vi "Generate 2D scan Waveform.vi"() -> ()   [LabVIEW 2014]
uses:
  <vilib>/Analysis/NI_AALBase.lvlib
  <vilib>/Analysis/1siggen.llb/Ramp Pattern by Samples.vi
  Controls/Translation Stage Types.ctl
  Hardware/Table Stage/Controls/Translation Stage Cluster.ctl
  Controls/System Parameters.ctl
panel:
  out "XY Graph":cluster{"X":dbl, "Y":dbl}[](graph)
  out "um/px":dbl
  in  "System Parameters [In]":T1={"Optical /HW Parameters"={"Focal Length [mm]"=0.0, "Scan Lens EFL[mm]"=0.0, "Tube Lens EFL[mm]"=0.0, "Galvo V Range (+/-)"=0.0, "Galvo Max Half Angle [Deg]"=0.0, "Max Galvo Range[%]"=0.0}, "Vibratome"={"Z Bottom [mm]"=0.0, "Pre Cut Dwell [s]"=0.0, "Blade Frequency [RPM]"=0, "Slice Speed [mm/s]"=0.0, "Post Cut Dwell [s]"=0.0, "Ramp Time [s]"=0.0, "Start X [mm]"=0.0, "Start Y [mm]"=0.0, "Slice Length [mm]"=0.0, "Slice Axis"=enum."Y Axis", "Controller VISA Ref"="COM4"}, "Table Stages"={"X Stage"={"Position"=0.0, "Is.Enabled?"=FALSE, "Is.Connected?"=FALSE, "Device SN"="45876539", "AccelerationMaximum"=0.0, "VelocityMaximum"=0.0, "Acceleration"=0.0, "Velocity"=0.0, "waitTimeout (ms)"=0, "Model"=enum."None", "Is.Homed?"=FALSE}, "Y Stage"={"Position"=0.0, "Is.Enabled?"=FALSE, "Is.Connected?"=FALSE, "Device SN"="45876539", "AccelerationMaximum"=0.0, "VelocityMaximum"=0.0, "Acceleration"=0.0, "Velocity"=0.0, "waitTimeout (ms)"=0, "Model"=enum."None", "Is.Homed?"=FALSE}, "Z Stage"={"Position"=0.0, "Is.Enabled?"=FALSE, "Is.Connected?"=FALSE, "Device SN"="45876539", "AccelerationMaximum"=0.0, "VelocityMaximum"=0.0, "Acceleration"=0.0, "Velocity"=0.0, "waitTimeout (ms)"=0, "Model"=enum."None", "Is.Homed?"=FALSE}}, "Imaging Parameter"={"Pixel Dwell Time [ms]"=0.0, "XY Center [um]"={"X"=1.0, "Y"=1.0}, "Zoom Factor"=1.0, "Display Channel"=enum."Channel A", "XY Image Resolution"=enum."256 x 256", "Custom"=FALSE, "Custom Size"={"X"=1, "Y"=1}, "Averaging"={"A Frame Ave."=1, "B Frame Ave."=1, "C Frame Ave. "=1}}} {"Imaging Parameter"."Custom Size"."Y" min=1 max=30 step=1; "Imaging Parameter"."Custom Size"."X" min=1 max=30 step=1; "Imaging Parameter"."XY Center [um]"."Y" min=1.0 max=30.0 step=1.0; "Imaging Parameter"."XY Center [um]"."X" min=1.0 max=30.0 step=1.0; "Imaging Parameter"."Averaging"."C Frame Ave." min=1 max=30 step=1; "Imaging Parameter"."Averaging"."B Frame Ave." min=1 max=30 step=1; "Imaging Parameter"."Averaging"."A Frame Ave." min=1 max=30 step=1; "Imaging Parameter"."Zoom Factor" min=1.0 max=10.0 step=0.1 scale=1.0..30.0; "Imaging Parameter"."Pixel Dwell Time [ms]" min=0.0 max=10.0 step=0.01}
  # "X"
  # "X"
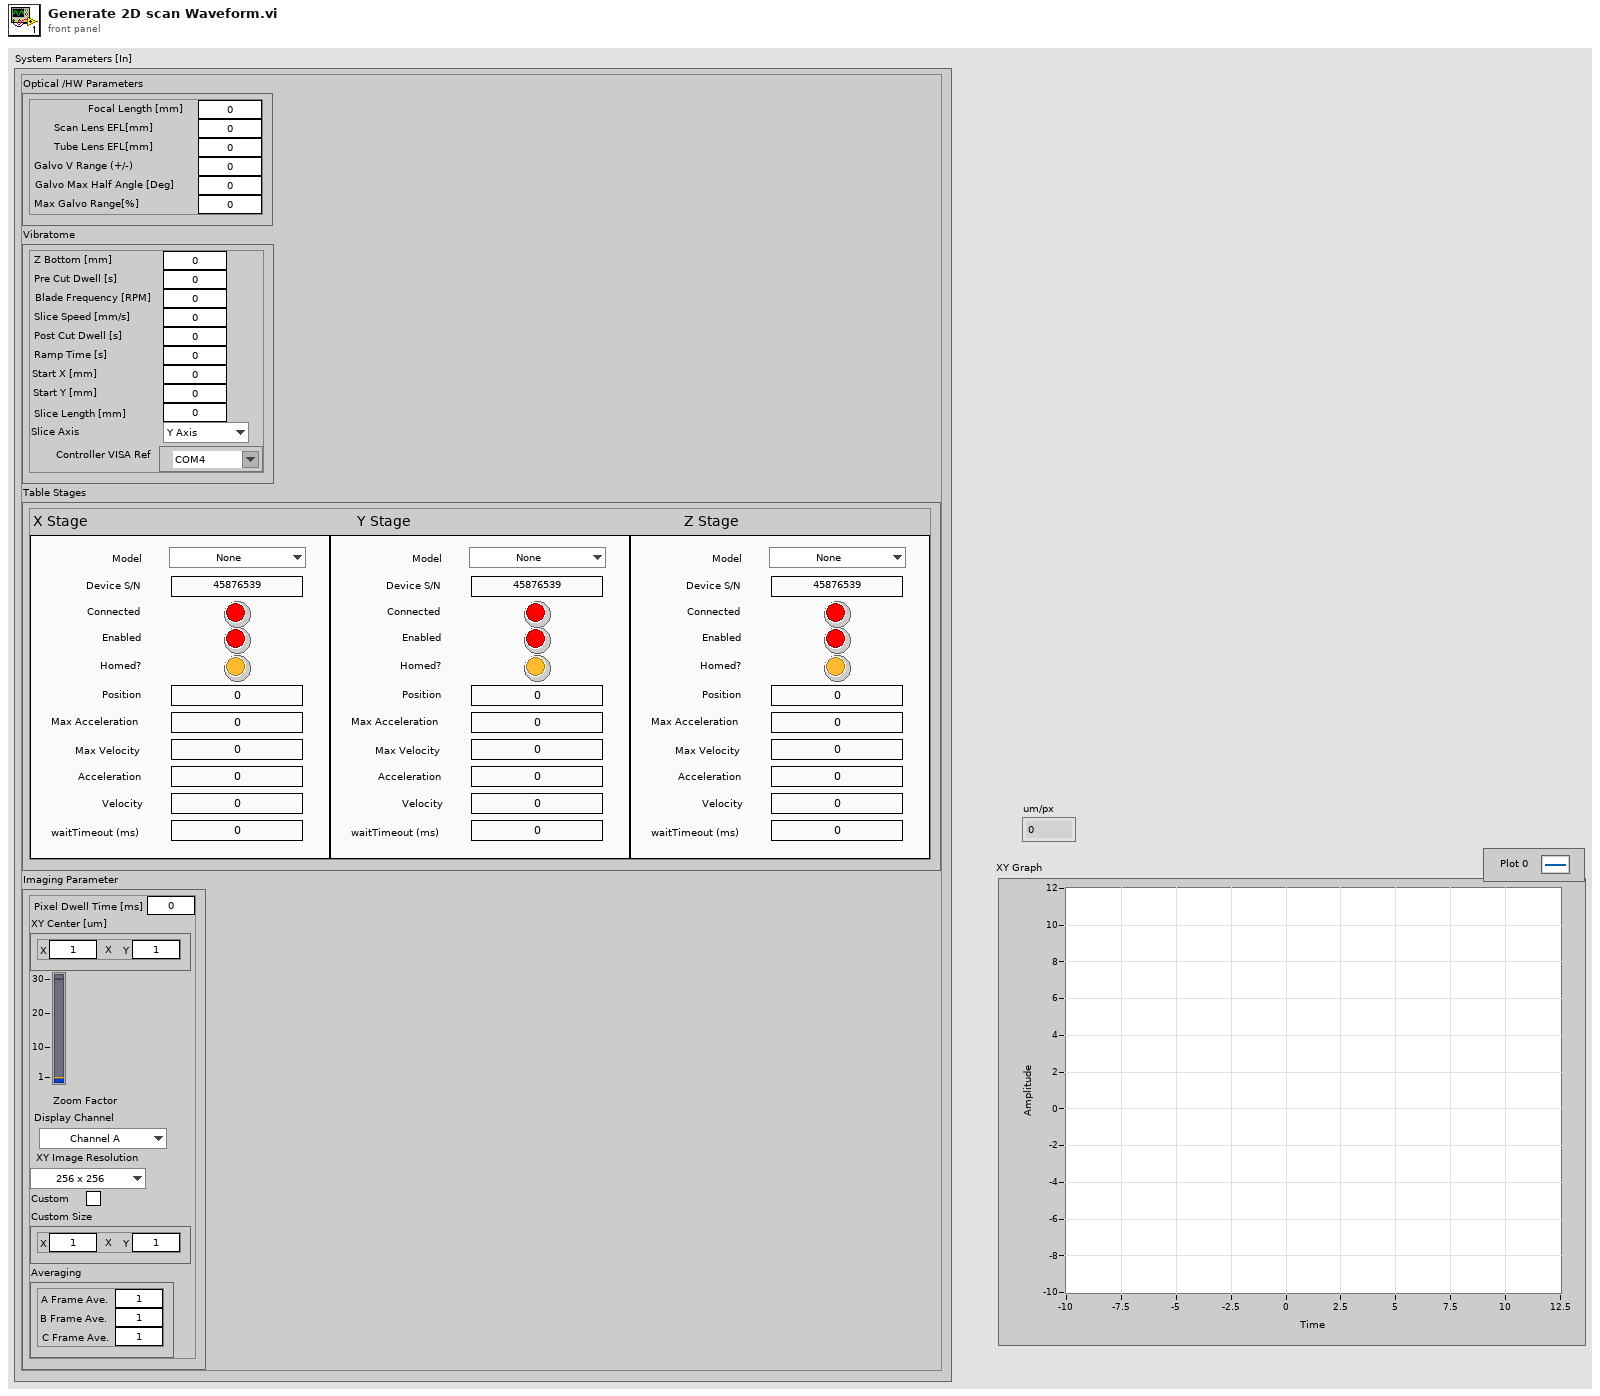
[diagram p1: front panel]
types:
  T1 = typedef "System Parameters.ctl" = cluster{"Optical /HW Parameters":cluster{"Focal Length [mm]":dbl, "Scan Lens EFL[mm]":dbl, "Tube Lens EFL[mm]":dbl, "Galvo V Range (+/-)":dbl, "Galvo Max Half Angle [Deg]":dbl, "Max Galvo Range[%]":dbl}, "Vibratome":cluster{"Z Bottom [mm]":dbl, "Pre Cut Dwell [s]":dbl, "Blade Frequency [RPM]":u16, "Slice Speed [mm/s]":dbl, "Post Cut Dwell [s]":dbl, "Ramp Time [s]":dbl, "Start X [mm]":dbl, "Start Y [mm]":dbl, "Slice Length [mm]":dbl, "Slice Axis":enum16{"X Axis", "Y Axis", "Z Axis"}, "Controller VISA Ref":refnum<visa-resource-name>}, "Table Stages":cluster{"X Stage":T2, "Y Stage":T2, "Z Stage":T2}, "Imaging Parameter":cluster{"Pixel Dwell Time [ms]":dbl, "XY Center [um]":cluster{"X":dbl, "Y":dbl}, "Zoom Factor":dbl, "Display Channel":enum16{"Channel A", "Channel B", "Channel A and B"}, "XY Image Resolution":enum16{"32 x 32", "64 x 64", "128 x 128", "256 x 256", "512 x 512", "1024 x 1024", "2048 x 2048"}, "Custom":bool, "Custom Size":cluster{"X":u16, "Y":u16}, "Averaging":cluster{"A Frame Ave.":u8, "B Frame Ave.":u8, "C Frame Ave. ":u8}}}
  T2 = typedef "Translation Stage Cluster.ctl" = cluster{"Position":dbl, "Is.Enabled?":bool, "Is.Connected?":bool, "Device SN":string, "AccelerationMaximum":dbl, "VelocityMaximum":dbl, "Acceleration":dbl, "Velocity":dbl, "waitTimeout (ms)":i32, "Model":T3, "Is.Homed?":bool}
  T3 = typedef "Translation Stage Types.ctl" = enum16{"None", "Thorlabs LTS", "Thorlabs MLJ"}
  T4 = cluster{"Pixel Dwell Time [ms]":dbl, "XY Center [um]":cluster{"X":dbl, "Y":dbl}, "Zoom Factor":dbl, "Display Channel":enum16{"Channel A", "Channel B", "Channel A and B"}, "XY Image Resolution":enum16{"32 x 32", "64 x 64", "128 x 128", "256 x 256", "512 x 512", "1024 x 1024", "2048 x 2048"}, "Custom":bool, "Custom Size":cluster{"X":u16, "Y":u16}, "Averaging":cluster{"A Frame Ave.":u8, "B Frame Ave.":u8, "C Frame Ave. ":u8}}
  T5 = enum16{"32 x 32", "64 x 64", "128 x 128", "256 x 256", "512 x 512", "1024 x 1024", "2048 x 2048"}
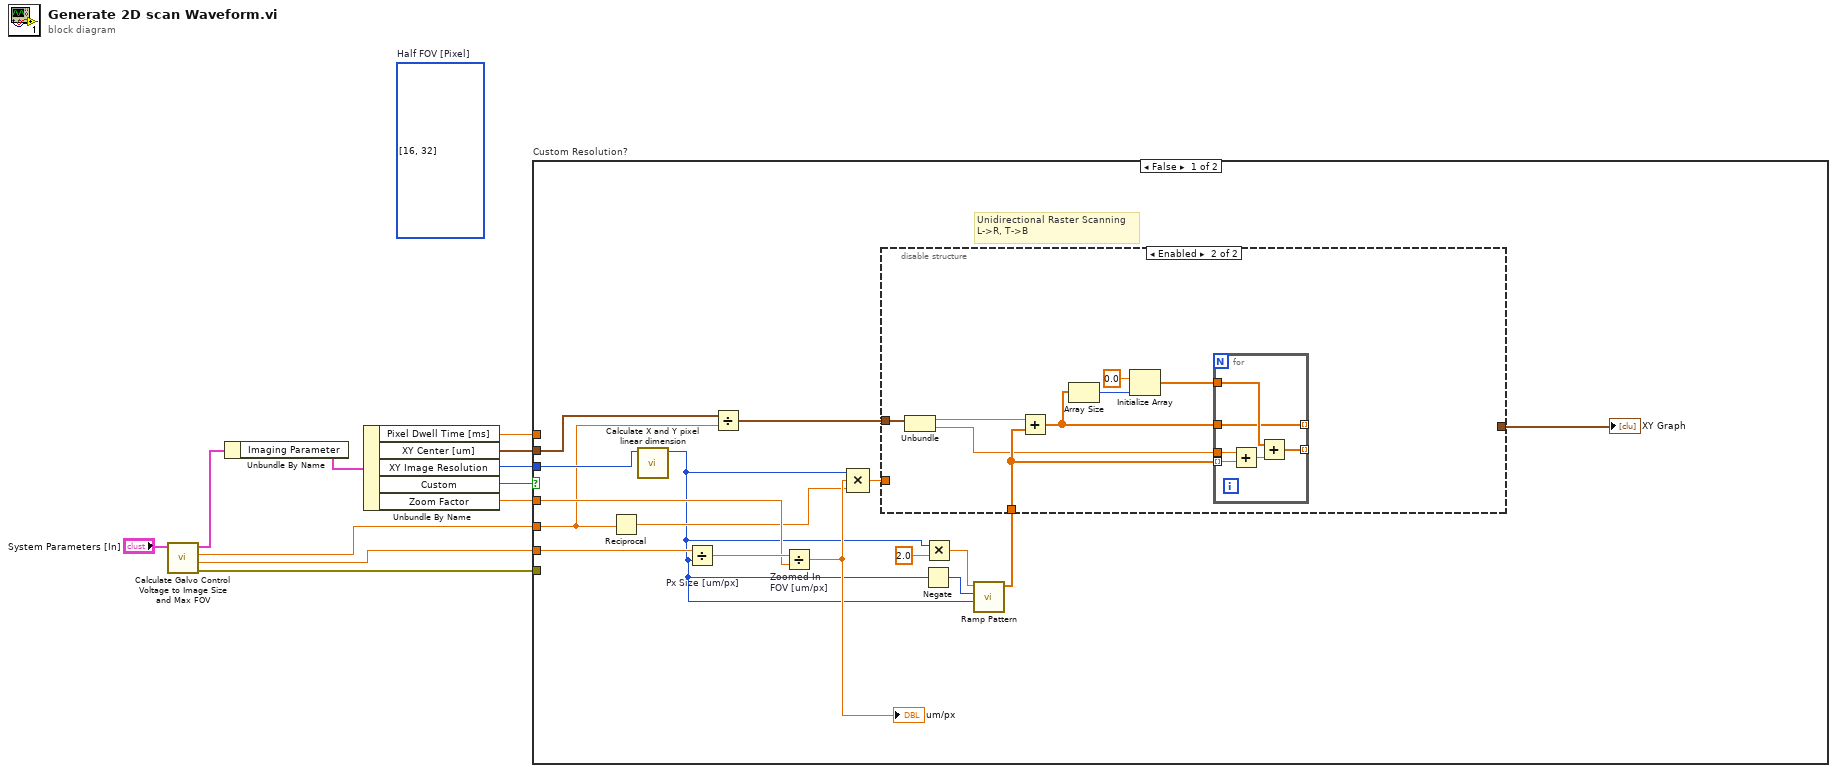
[diagram p0: block diagram]
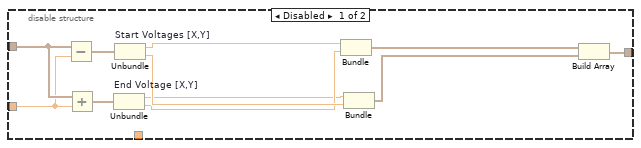
[diagram p2: hidden frame]
diagram:
  (unwired) i32[] [16, 32]  # Half FOV [Pixel]
  n1 = call "Calculate Galvo Control Voltage to Image Size and Max FOV.vi"("System Parameters [In]"="System Parameters [In]") -> ("Error Out"=w3:errorcluster, "Max Half FOV (um)"=w2:dbl, "Galvo [um/V]"=w1:dbl, "System Parameters [Out]"=w7:T1)  [unwired: 7 in]
  n2 = Unbundle By Name(w7) -> ("Imaging Parameter"=w11:T4)
  n3 = Unbundle By Name(w11) -> ("Pixel Dwell Time [ms]"=w4:dbl, "XY Center [um]"=w9:cluster{"X":dbl, "Y":dbl}, "XY Image Resolution"=w5:T5, "Custom"=w6:bool, "Zoom Factor"=w10:dbl)
  n4 = case "Custom Resolution?" shown="False" w6 {
    tunnel: w10 -> [w22 _]
    tunnel: w9 -> [w27 _]
    tunnel: w5 -> [w26 _]
    tunnel: w4 -> [_ _]
    tunnel: w3 -> [_ _]
    tunnel: w2 -> [w24 _]
    tunnel: w1 -> [w18 _]
    frame False {
      # "Unidirectional Raster Scanning\nL->R, T->B"
      n5 = Reciprocal(x=w18) -> (1/x=w17:dbl)
      n6 = call "Calculate X and Y pixel linear dimension.vi"("XY Image Resolution"=w26) -> ("X Px Dim (HFOV)"=w13:u16)  [unwired: 7 in, 3 out]
      n7 = Divide "Px Size [um/px]"(x=w24, y=w13) -> (x/y=w23:dbl)
      n8 = Divide(x=w27, y=w18) -> (x/y=w25:cluster{"X":dbl, "Y":dbl})
      n9 = Divide "Zoomed In\nFOV [um/px]"(x=w23, y=w22) -> (x/y=w20:dbl)
      "um/px" <- w20
      n10 = Compound Arithmetic op=MULTIPLY(w13, w20, w17) -> (w19:dbl)
      n11 = Negate(x=w13) -> (-x=w14:i16)
      n12 = Multiply(x=w13, y=2.0) -> (x*y=w15:dbl)
      n13 = call-poly <vilib>:"Ramp Pattern.vi"("start"=w13, "end"=w14, "samples"=w15) -> ("Ramp Pattern"=w12:dbl[])  [unwired: 7 in, 1 out]
      n14 = disable-structure shown="Enabled" {
        disable-tunnel: w25 -> [w38 w46]
        disable-tunnel: [w31 _] -> w21
        disable-tunnel: w19 -> [w30 _]
        disable-tunnel: w12 -> [_ w44]
        frame Disabled {
          n15 = Subtract(x=w38, y=w30) -> (x-y=w37:cluster{"X":dbl, "Y":dbl})
          n16 = Add(x=w38, y=w30) -> (x+y=w36:cluster{"X":dbl, "Y":dbl})
          n17 = Unbundle "End Voltage [X,Y]"(w36) -> ("X"=w28:dbl, "Y"=w34:dbl)
          n18 = Unbundle "Start Voltages [X,Y]"(w37) -> ("X"=w29:dbl, "Y"=w35:dbl)
          n19 = Bundle("X"=w29, "Y"=w34) -> (w33:cluster{"X":dbl, "Y":dbl})  [unwired: 1 in]
          n20 = Bundle("X"=w28, "Y"=w35) -> (w32:cluster{"X":dbl, "Y":dbl})  [unwired: 1 in]
          n21 = Build Array(w33, w32) -> (w31:cluster{"X":dbl, "Y":dbl}[])
        }
        frame Enabled {
          n22 = Unbundle(w46) -> ("X"=w45:dbl, "Y"=w43:dbl)
          n23 = Add(x=w45, y=w44) -> (x+y=w41:dbl[])
          n24 = Array Size(array=w41) -> (size(s)=w42:i32)
          n25 = Initialize Array(0.0 ("element"), w42) -> (w39:dbl[])
          n26 = for {
            tunnel: w44 -> [w52] mode=indexing
            tunnel: w41 -> [w48]
            tunnel: w43 -> [w51]
            tunnel: w39 -> [w49]
            tunnel: [w48] -> _ mode=indexing
            tunnel: [w47] -> _ mode=indexing
            n27 = Add(x=w51, y=w52) -> (x+y=w50:dbl)
            n28 = Add(x=w49, y=w50) -> (x+y=w47:dbl[])
          }
        }
      }
      "XY Graph" <- w21
    }
    frame True {
    }
  }
